vi "Byte_data_변환(2).vi"() -> ()   [LabVIEW 2017]
panel:
  out "Unpack(4byte)_소수":sgl
  out "문자열":string
  out "숫자형 컨트롤 2":i32
  out "unsigned byte array":u8[][](array[numeric])
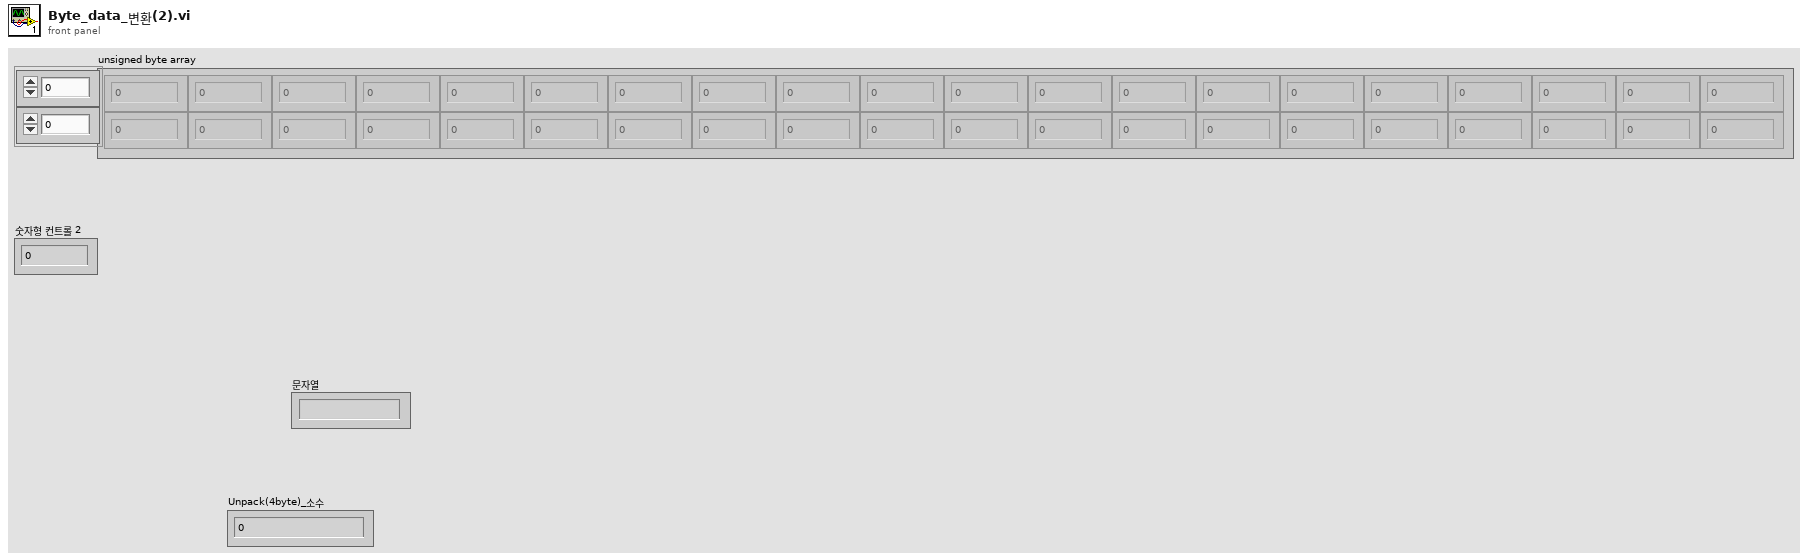
[diagram p1: front panel]
types:
  T1 = enum16{"Standard", "Buffered", "CRLF", "Immediate"}
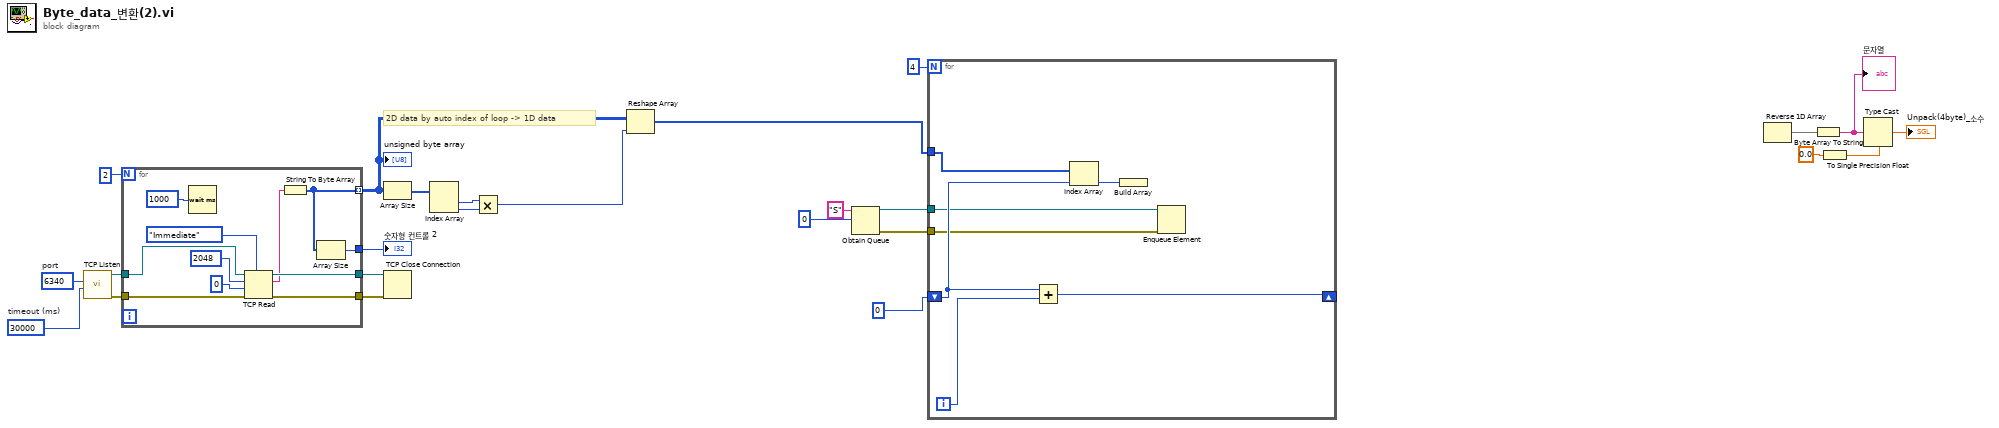
[diagram p0: block diagram]
diagram:
  w21 = u16 6340  # port
  w20 = 30000  # timeout (ms)
  # "2D data by auto index of loop -> 1D data"
  n1 = call <vilib>:"TCP Listen.vi"("timeout ms (wait forever: -1)"=w20, "port"=w21) -> ("error out"=w24:errorcluster, "connection ID"=w25:refnum<k5>)  [unwired: 5 in, 3 out]
  n2 = for {
    N: 2 -> [_]
    tunnel: w25 -> [w36]
    tunnel: w24 -> [w35]
    tunnel: [w34] -> w23
    tunnel: [w33] -> w22
    tunnel: [w28] -> w15 mode=indexing
    tunnel: [w27] -> w8
    n3 = Wait (ms)(milliseconds to wait=u32 1000 ("대기 시간 (ms)")) -> ()  [unwired: 1 out]
    n4 = TCP Read(connection ID=w36, bytes to read=2048 ("읽을 바이트"), error in (no error)=w35, 7:T1."Immediate" ("모드(standard)"), 9:0 ("타임아웃 ms (25000)")) -> (connection ID out=w34:refnum<k5>, data out=w26:string, error out=w33:errorcluster)
    n5 = String To Byte Array(string=w26) -> (unsigned byte array=w28:u8[])
    n6 = Array Size(array=w28) -> (size(s)=w27:i32)
  }
  "unsigned byte array" <- w15
  "숫자형 컨트롤 2" <- w8
  n7 = Array Size(array=w15) -> (size(s)=w16:i32[])
  n8 = TCP Close Connection(connection ID=w23, error in (no error)=w22) -> ()  [unwired: 3 out]
  n9 = Index Array(array=w16) -> (element #1=w18:i32, element #2=w17:i32)  [unwired: 2 in]
  n10 = Multiply(x=w18, y=w17) -> (x*y=w19:i32)
  n11 = Reshape Array(w15, w19) -> (w6:u8[])
  n12 = Obtain Queue(name (unnamed)="S" ("이름(이름없음)"), element data type=0) -> (queue out=w2:refnum<queue>, error out=w1:errorcluster)  [unwired: 3 in, 1 out]
  n13 = for {
    N: 4 -> [_]
    tunnel: w6 -> [w43]
    shift-right: [w40] -> _
    shift-left: 0 -> [w42]
    tunnel: w2 -> [w38]
    tunnel: w1 -> [w37]
    i -> [w41]
    n14 = Add(x=w42, y=w41) -> (x+y=w40:i32)
    n15 = Index Array(array=w43, index=w42) -> (element=w39:u8)
    n16 = Build Array(w39) -> ()  [unwired: 1 out]
    n17 = Enqueue Element(queue=w38, error in (no error)=w37) -> ()  [unwired: 2 in, 3 out]
  }
  n18 = Reverse 1D Array() -> (reversed array=w10:dbl[])  [unwired: 1 in]
  n19 = Byte Array To String(unsigned byte array=w10) -> (string=w11:string)
  "문자열" <- w11
  n20 = To Single Precision Float(number=0.0) -> (single precision float=w13:sgl)
  n21 = Type Cast(type=w13, x=w11) -> (*(type *) &x=→"Unpack(4byte)_소수":sgl)
